vi "ChipKit Thumbstick.vi"() -> ()   [LabVIEW 2011, in "LabVIEW Interface for ChipKit.lvlib"]
doc: "An example that uses an ChipKit to capture input from an analog thumb stick which is used to generate colors based on the angle and magnitude of the thumb stick. These colors are displayed on the front panel and sent to an RGB LED . (The RGB LED can easily be replaced with BlinkMs)"
uses:
  vi.lib/LabVIEW Interface for ChipKit/LabVIEW Interface for ChipKit.lvlib
panel:
  in  "VISA resource name":refnum<visa-resource-name>
  out "Color":u32(colorbox)=1297
  out "Vertical Axis":dbl(slide)=2.3226 scale=0.0..5.0
  out "Horizontal Axis":dbl(slide)=2.3863 scale=0.0..5.0
  in  "Stop":bool
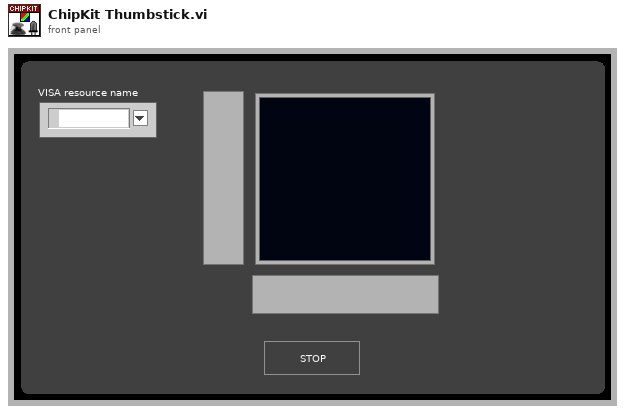
[diagram p1: front panel]
types:
  T1 = typedef "LabVIEW Interface for ChipKit.lvlib/Chipkit Resource.ctl" = cluster{"VISA resource":refnum<visa-resource-name>, "Board Type":T2, "Connection Type":enum8{"USB / Serial"}, "Bytes Per Packet (15)":u8}
  T2 = typedef "LabVIEW Interface for ChipKit.lvlib/Board Type.ctl" = enum16{"Arduino Uno", "Dimuelanove w/Atmega 328", "Mega 2560", "Chipkit Uno32", "Chipkit Max32"}
  T3 = cluster{"Horizontal Axis Pin":dbl, "Vertical Axis Pin":dbl, "Select Pin":dbl}
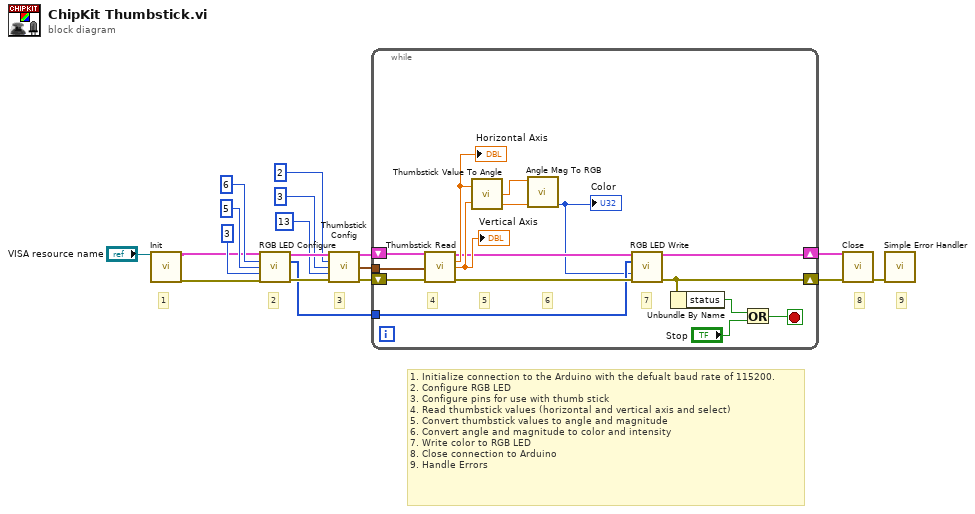
[diagram p0: block diagram]
diagram:
  # "9"
  # "8"
  # "3"
  # "2"
  # "1"
  # "1. Initialize connection to the Arduino with the defualt baud rate of 115200.\n2. Configure RGB LED\n3. Configure pins for use with thumb stick\n4. Read thumbstick values (horizontal and vertical axis and select)\n5. Convert thumbstick values to angle and magnitude\n6. Convert angle and magnitude to color and intensity\n7. Write color to RGB LED\n8. Close connection to Arduino\n9. Handle Errors"
  n1 = call "Init.vi"("VISA resource"="VISA resource name") -> ("Arduino Resource"=w3:T1, "error out"=w2:errorcluster)  [unwired: 17 in]
  n2 = call "RGB LED Configure.vi"("Arduino Resource"=w3, "Red Pin"=u8 6, "Green Pin"=u8 5, "Blue Pin"=u8 3, "error in"=w2) -> ("Arduino Resource"=w13:T1, "RGB LED Pins"=w4:u8[], "error out"=w12:errorcluster)  [unwired: 8 in]
  n3 = call "Thumbstick Config.vi"("Arduino Resource"=w13, "Horizontal Axis AI Pin"=u8 2, "Vertical Axis AI Pin"=u8 3, "Select DI Pin"=u8 13, "error in"=w12) -> ("Arduino Resource"=w17:T1, "Thumbstick Data"=w18:T3, "error out"=w16:errorcluster)  [unwired: 8 in]
  n4 = while {
    shift-right: [w20] -> w6
    shift-left: w17 -> [w34]
    shift-right: [w19] -> w15
    shift-left: w16 -> [w33]
    tunnel: w18 -> [w32]
    tunnel: w4 -> [w22]
    stop <- w24 stop-if-true
    # "7"
    # "6"
    # "5"
    # "4"
    n5 = call "Thumbstick Read.vi"("Arduino Resource"=w34, "Thumbstick Data"=w32, "error in"=w33) -> ("Arduino Resource"=w23:T1, "Horizontal Axis"=w29:dbl, "Vertical Axis"=w28:dbl, "error out"=w27:errorcluster)  [unwired: 8 in, 1 out]
    "Horizontal Axis" <- w29
    "Vertical Axis" <- w28
    n6 = call "Thumbstick Value To Angle.vi"("Vertical Axis"=w28, "Horizontal Axis"=w29) -> ("Magnitude"=w31:dbl, "Degrees"=w30:dbl)  [unwired: 1 out]
    n7 = call "Angle Mag To RGB.vi"("Magnitude (0-1)"=w31, "Angle (Degrees)"=w30) -> ("RGB Color"=w21:u32)  [unwired: 6 in, 3 out]
    "Color" <- w21
    n8 = call "RGB LED Write.vi"("Arduino Resource"=w23, "RGB LED Pins"=w22, "Color"=w21, "error in"=w27) -> ("Arduino Resource"=w20:T1, "error out"=w19:errorcluster)  [unwired: 9 in, 1 out]
    n9 = Unbundle By Name(w19) -> ("status"=w26:bool)
    n10 = Or(x=w26, y="Stop") -> (x .or. y?=w24:bool)
  }
  n11 = call "Close.vi"("Arduino Resource"=w6, "error in"=w15) -> ("error out"=w14:errorcluster)  [unwired: 13 in]
  n12 = call <vilib>:"Simple Error Handler.vi"("error in (no error)"=w14) -> ()  [unwired: 4 in, 5 out]
